vi "总磷启动(子VI).vi"(11 "元素":T1(ring)) -> (0 "error out":T2={"status"=FALSE, "代码"=4, "source"=""} caption="错误输出" {"代码" items=["执行成功"=1, "执行失败，但不知道原因"=2, "命令请求条件错误"=3, "通讯超时"=4, "系统繁忙不能执行"=5, "系统故障"=6, "没有数据"=100]})   [LabVIEW 2016]
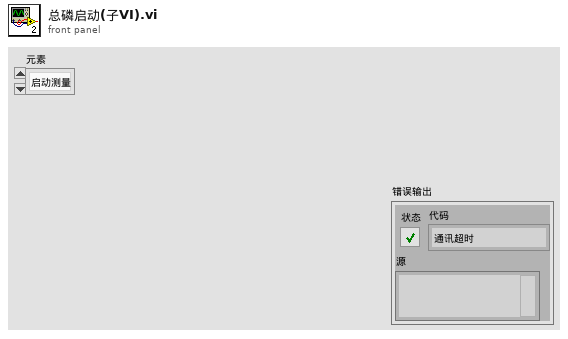
[diagram p1: front panel]
types:
  T1 = enum16{"启动测量", "标样核查", "零点核查", "跨度核查", "空白测试", "平行样测试", "加标回收", "空白校准", "标样校准", "初始化（清洗）", "停止测试", "仪器重启", "校时", "模式设置", "测量间隔设置"}
  T2 = cluster{"status":bool, "代码":u16, "source":string}
  T3 = enum16{"空闲", "水样测试", "标样核查", "零点核查", "跨度核查", "空白测试", "平行样测试", "加标回收", "空白校准", "标样校准", "初始化（清洗）"}
  T4 = cluster{"系统时间":timestamp, "工作状态":u16, "测量模式":enum16{"待机", "连续模式", "周期模式", "定点模式", "受控模式", "手动模式"}, "告警代码":u16, "故障代码":u16, "日志代码":u16, "软件版本":u16, "F0":sgl, "F1":sgl, "F2":sgl, "F3":sgl, "T":sgl, "H":sgl, "id":u16, "flowid":u16, "量程":u16, "总磷控温温度1":sgl, "营养盐控温温度2":sgl, "ADC":sgl}
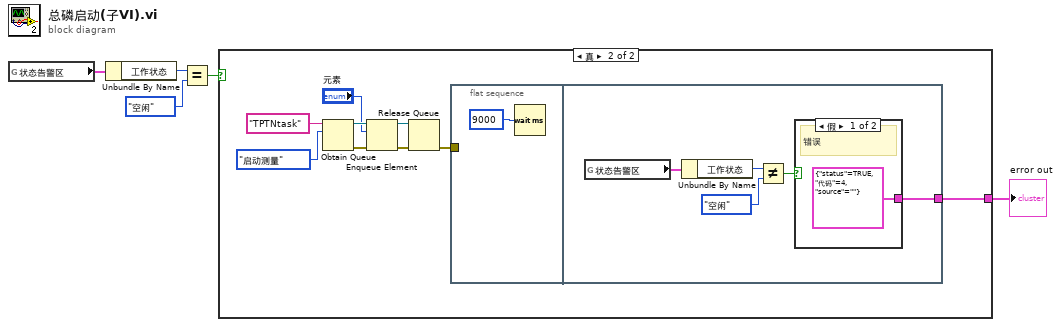
[diagram p0: block diagram]
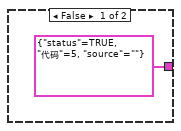
[diagram p2: hidden frame]
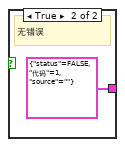
[diagram p3: hidden frame]
diagram:
  n1 = global read "VAR总磷总氮全局变量.vi" "状态告警区"() -> (w2:T4)
  n2 = Unbundle By Name(w2) -> ("工作状态"=w5:u16)
  n3 = Equal?(x=w5, y=T3."空闲") -> (x = y?=w3:bool)
  n4 = case shown="真" w3 {
    tunnel: [T2 {"status"=TRUE, "代码"=5, "source"=""} ("error out") w12] -> w1
    frame False {
    }
    frame True {
      n5 = Obtain Queue(name (unnamed)="TPTNtask" ("名称（未命名）"), element data type=T1."启动测量" ("控制命令")) -> (queue out=w9:refnum<queue>, error out=w8:errorcluster)  [unwired: 3 in, 1 out]
      n6 = Enqueue Element(queue=w9, element="元素", error in (no error)=w8) -> (queue out=w15:refnum<queue>, error out=w14:errorcluster)  [unwired: 1 in, 1 out]
      n7 = Release Queue(queue=w15, error in (no error)=w14) -> (error out=w13:errorcluster)  [unwired: 1 in, 2 out]
      n8 = flat-sequence {
        tunnel: w13 -> [_]
        tunnel: [w21] -> w12
        frame #0 {
          n9 = Wait (ms)(milliseconds to wait=u32 9000 ("等待时间（毫秒）")) -> ()  [unwired: 1 out]
        }
        frame #1 {
          n10 = global read "VAR总磷总氮全局变量.vi" "状态告警区"() -> (w17:T4)
          n11 = Unbundle By Name(w17) -> ("工作状态"=w19:u16)
          n12 = Not Equal?(x=w19, y=T3."空闲") -> (x != y?=w18:bool)
          n13 = case shown="假" w18 {
            tunnel: [T2 {"status"=TRUE, "代码"=4, "source"=""} ("error out") T2 {"status"=FALSE, "代码"=1, "source"=""} ("error out")] -> w21
            frame False {
              # "错误"
            }
            frame True {
              # "无错误"
            }
          }
        }
      }
    }
  }
  "error out" <- w1
